vi "Marshal.vi"(8 "error in (no error)":errorcluster, 11 "int32 in":refnum<class "sint64.lvclass">) -> (0 "error out":errorcluster, 2 "Buffer":u8[](array[numeric]), 3 "int32 out":refnum<class "sint64.lvclass">)   [LabVIEW 2020, in "Protobuf RAW.lvlib" / "sint64.lvclass"]
uses:
  sint64.lvclass
  sint64.lvclass/sint64.ctl
  f710cda7-38bf-45a5-8a40-040cea5f9839.vi
  4736b2cc-328e-48c1-834c-9aec0f57f3c9.vi
  f710cda7-38bf-45a5-8a40-040cea5f9839.vi/45576c96-348a-4a29-82b0-147ecb2792d1.vi
  4736b2cc-328e-48c1-834c-9aec0f57f3c9.vi/0f065a35-b637-42bd-ae45-04c3465bdb97.vi
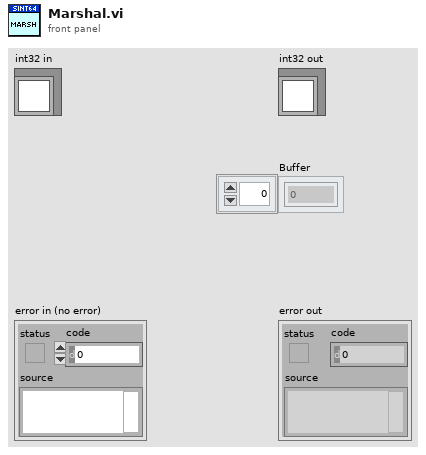
[diagram p1: front panel]
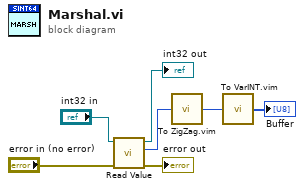
[diagram p0: block diagram]
diagram:
  n1 = call "Read Value.vi"("error in (no error)"="error in (no error)", "int32 in"="int32 in") -> ("error out"=→"error out":errorcluster, "Value"=w1:i64, "int32 out"=→"int32 out":refnum<class "sint64.lvclass">)  [unwired: 7 in]
  n2 = call "To ZigZag.vim"("Signed Integer"=w1) -> ("Zig Zag"=w6:u64)
  n3 = call "To VarINT.vim"("Integer"=w6) -> ("LEB128"=→"Buffer":u8[])
